vi "Logging Format Tree Entry.vi"() -> ()   [LabVIEW 2012, in "femtoRoboLib.lvlib"]
uses:
  Controls/Log Entry.ctl
  Controls/Log Value Type.ctl
  Controls/Log Value Cluster.ctl
  femtoRoboLib.lvlib
panel:
  out "Entry String":string[](array[string])
  in  "Name":string
  in  "Entries":T1[](array[typedef])
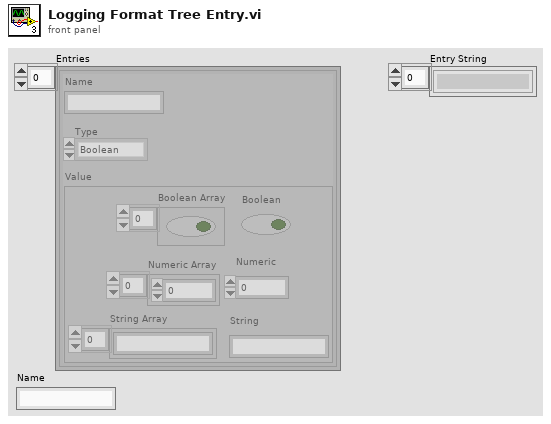
[diagram p1: front panel]
types:
  T1 = typedef "femtoRoboLib.lvlib/Log Entry.ctl" = cluster{"Name":string, "Type":T2, "Value":T3}
  T2 = typedef "femtoRoboLib.lvlib/Log Value Type.ctl" = enum16{"Boolean", "Numeric", "String", "Boolean Array", "Numeric Array", "String Array"}
  T3 = typedef "femtoRoboLib.lvlib/Log Value Cluster.ctl" = cluster{"Boolean Array":bool[], "Boolean":bool, "Numeric Array":dbl[], "Numeric":dbl, "String Array":string[], "String":string}
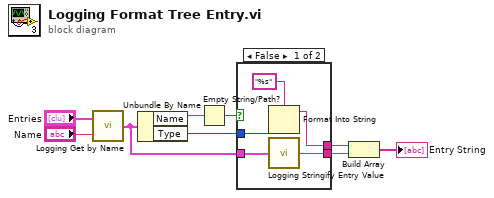
[diagram p0: block diagram]
diagram:
  n1 = call "Logging Get by Name.vi"("Name"="Name", "Entries"="Entries") -> ("Entry"=w8:T1)
  n2 = Unbundle By Name(w8) -> ("Name"=w4:string, "Type"=w9:T2)
  n3 = Empty String/Path?(string/path=w4) -> (empty?=w5:bool)
  n4 = case shown="False" w5 {
    tunnel: w9 -> [w13 _]
    tunnel: w8 -> [w12 _]
    tunnel: [w11 _] -> w2
    tunnel: [w10 _] -> w1
    frame False {
      n5 = Format Into String(format string="%s", w13) -> (resulting string=w11:string)  [unwired: 2 in, 1 out]
      n6 = call "Logging Stringify Entry Value.vi"("Entry"=w12) -> ("String"=w10:string)
    }
    frame True {
    }
  }
  n7 = Build Array(w2, w1) -> (→"Entry String":string[])
